vi "RS232_Init.vi"(5 "error in (no error)":errorcluster) -> (14 "object out":refnum<class "RS232.lvclass">, 19 "error out":errorcluster)   [LabVIEW 2019, in "RS232.lvclass"]
uses:
  RS232.lvclass
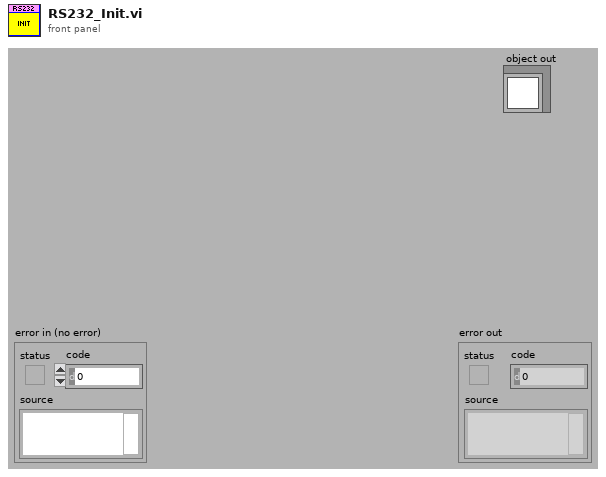
[diagram p1: front panel]
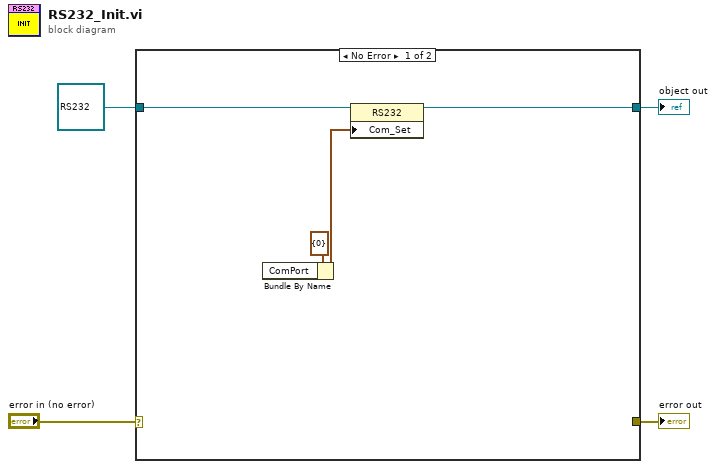
[diagram p0: block diagram]
diagram:
  n1 = case shown="No Error" "error in (no error)" {
    selector: "error in (no error)" -> [_ w10]
    tunnel: [w7 w11] -> w4
    tunnel: refnum<class "RS232.lvclass"> refnum ("object in") -> [w8 w11]
    tunnel: [w9 w10] -> w1
    frame No Error {
      n2 = Bundle By Name(cluster=cluster{"ComPort":u16} {"ComPort"=0} ("Com_Set")) -> (w5:cluster{"ComPort":u16})  [unwired: 1 in]
      n3 = property class="RS232"(reference=w8, "Com_Set"=w5) -> (reference out=w7:refnum<class "RS232.lvclass">)  [unwired: 1 in, 1 out]
    }
    frame Error {
    }
  }
  "object out" <- w4
  "error out" <- w1
